vi "4R serial robot 3D simulation.vi"() -> ()   [LabVIEW 2014]
doc: "This example shows a robotic arm with four revolute joints (a 4R serial robot), and demonstrates how to use custom equations to deterministically compute inverse kinematics for the arm."
uses:
  <vilib>/Platform/TimedLoop/XDataNode/timing_clust.ctl
  <vilib>/Platform/TimedLoop/XDataNode/nitl_modes.ctl
  <vilib>/Platform/TimedLoop/XDataNode/wakeup.ctl
  <vilib>/robotics/Kinematics/Plotting/Tree Element.ctl
  <vilib>/robotics/Kinematics/Plotting/Element Type.ctl
  <vilib>/robotics/Kinematics/Plotting/Joint Type.ctl
  <vilib>/Utility/AngleManip/Degrees to Radians (Scalar DBL).vi
  <vilib>/Platform/TimedLoop/XDataNode/XDataNode.xnode
  <vilib>/robotics/Kinematics/Plotting/NI_Robotics_3DKinematics.lvlib
  <vilib>/Platform/TimedLoop/XDataNode/XDNodeRunTimeDep.lvlib
  <vilib>/Utility/AngleManip/NI_AngleManipulation.lvlib
panel:
  out "Invalid Position":bool
  in  "Joint angles":dbl[](array[numeric])
  in  "Y":dbl(slide)=4.790575916230366 scale=-5.0..12.0
  in  "X":dbl(slide)=4.08910891089109 scale=-5.0..12.0
  in  "theta":dbl(knob) scale=-180.0..180.0
  in  "stop":bool
  out "3D Picture Control":refnum<vi>(3d-picture)
  # "This example shows a robotic arm with four revolute joints (a 4R serial robot), and demonstrates how to use custom equations to deterministically compute inverse kinematics for the arm.\n\nUse the X and Y sliders to move the end effector, and the dial to set the rotation of the base. This VI uses inverse kinematics to compute the positions and angles of the joints."
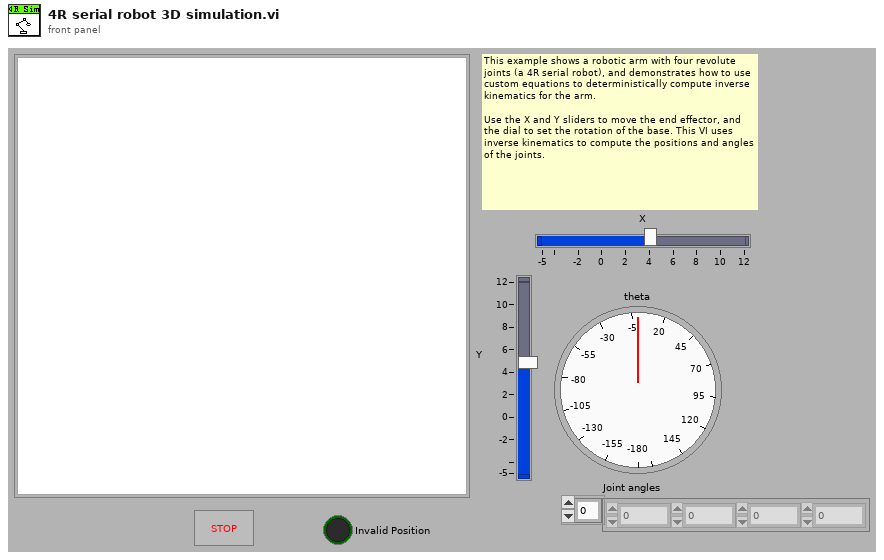
[diagram p1: front panel]
types:
  T1 = typedef "NI_Robotics_3DKinematics.lvlib/Tree Element.ctl" = cluster{"Name":string, "Parent":string, "Type":T2, "Visible?":bool, "Geometry Definition":dbl[], "Position WRT Parent (X,Y,Z)":dbl[], "Rotation WRT Parent (degrees)":dbl[], "Joint Type":T3, "Geometry File Path":path, "Indent Level":i32, "Color":u32}
  T2 = typedef "NI_Robotics_3DKinematics.lvlib/Element Type.ctl" = enum16{"Joint", "Box", "Cylinder", "Cone", "Sphere", "ASE File", "VRML File", "STL File", "Space"}
  T3 = typedef "NI_Robotics_3DKinematics.lvlib/Joint Type.ctl" = enum16{"Trans_X", "Trans_Y", "Trans_Z", "Rot_X", "Rot_Y", "Rot_Z", "None"}
  T4 = typedef "XDNodeRunTimeDep.lvlib/timing_clust.ctl" = cluster{"Expected End [f-1]":u64, "Actual End [f-1]":u64, "Finished Late? [f-1]":bool, "Expected End [i-1]":u64, "Actual End [i-1]":u64, "Finished Late? [i-1]":bool, "Expected Start [i]":u64, "Actual Start [i]":u64, "Expected Start [f]":u64, "Actual Start [f]":u64, "Source Name":string, "Structure Name":string, "Period":i64, "Deadline":i64, "Offset":i64, "Start":i64, "Priority":i32, "Timeout":i32, "Mode":T5, "Wakeup Reason":T6, "Error":errorcluster, "Source Type":string, "Secondary Source Type":string, "Global End Time":u64, "Global Start Time":u64, "Frame Duration":u64, "Iteration Duration":u64, "Assigned CPU":i32, "I/O Scan Engine Mode":u32}
  T5 = typedef "XDNodeRunTimeDep.lvlib/nitl_modes.ctl" = enum32{"No Change", "Process missed periods, maintain original phase", "Discard missed periods, maintain original phase", "Process missed periods, ignore original phase", "Discard missed periods, ignore original phase"}
  T6 = typedef "XDNodeRunTimeDep.lvlib/wakeup.ctl" = enum32{"Normal", "Aborted", "Asynchronous wakeup", "Timing source error", "Timed loop error", "Timeout"}
  T7 = typedef "NI_Robotics_3DKinematics.lvlib/Joint Control.ctl" = cluster{"Joint Refnum":refnum<vi>, "Joint Type":T3, "Position WRT Parent":dbl[], "Rotation WRT Parent":dbl[], "Bar Refnum":refnum<vi>}
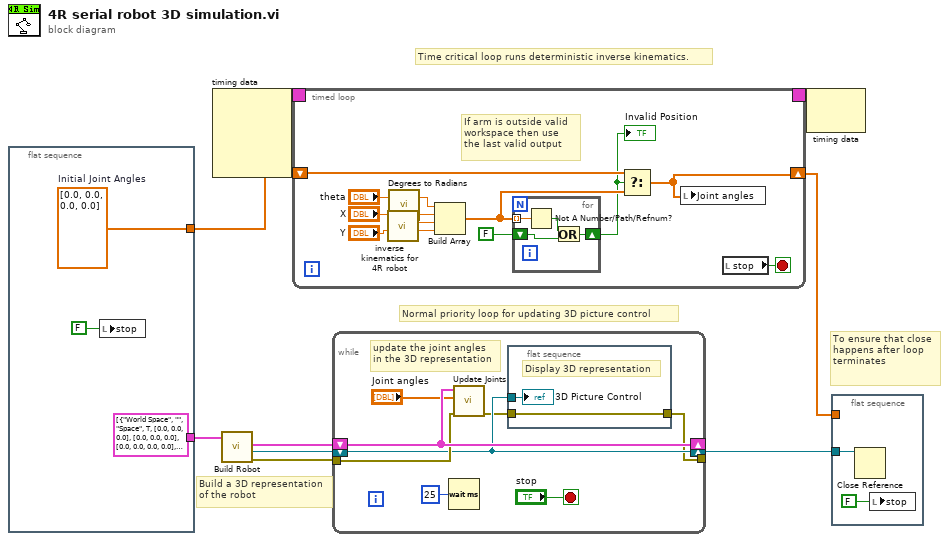
[diagram p0: block diagram]
diagram:
  # "To ensure that close happens after loop terminates"
  # "Build a 3D representation\nof the robot"
  # "Normal priority loop for updating 3D picture control"
  # "Time critical loop runs deterministic inverse kinematics."
  n1 = flat-sequence {
    tunnel: [w12] -> w3
    tunnel: [T1[] [{"Name"="World Space", "Parent"="", "Type"=enum."Space", "Visible?"=TRUE, "Geometry Definition"=[0.0, 0.0, 0.0], "Position WRT Parent (X,Y,Z)"=[0.0, 0.0, 0.0], "Rotation WRT Parent (degrees)"=[0.0, 0.0, 0.0, 0.0], "Joint Type"=enum."None", "Geometry File Path"=path "", "Indent Level"=0, "Color"=16711680}, {"Name"="Base", "Parent"="World Space", "Type"=enum."Cylinder", "Visible?"=TRUE, "Geometry Definition"=[1.0, 1.0, 1.0], "Position WRT Parent (X,Y,Z)"=[0.0, 0.5, 0.0], "Rotation WRT Parent (degrees)"=[1.0, 0.0, 0.0, 90.0], "Joint Type"=enum."None", "Geometry File Path"=path "", "Indent Level"=1, "Color"=16777224}, {"Name"="Joint 1", "Parent"="World Space", "Type"=enum."Joint", "Visible?"=TRUE, "Geometry Definition"=[0.0, 0.0, 0.0], "Position WRT Parent (X,Y,Z)"=[0.0, 1.0, 0.0], "Rotation WRT Parent (degrees)"=[0.0, 0.0, 0.0, 90.0], "Joint Type"=enum."Rot_Y", "Geometry File Path"=path "", "Indent Level"=1, "Color"=16711680}, {"Name"="Joint 3", "Parent"="Joint 1", "Type"=enum."Joint", "Visible?"=TRUE, "Geometry Definition"=[0.0, 0.0, 0.0], "Position WRT Parent (X,Y,Z)"=[0.0, 0.0, 0.0], "Rotation WRT Parent (degrees)"=[0.0, 0.0, 1.0, -90.0], "Joint Type"=enum."Rot_Z", "Geometry File Path"=path "", "Indent Level"=2, "Color"=16711680}, {"Name"="Link 1 A", "Parent"="Joint 3", "Type"=enum."Box", "Visible?"=TRUE, "Geometry Definition"=[0.9, 5.0, 0.5], "Position WRT Parent (X,Y,Z)"=[0.0, 2.0, 0.5], "Rotation WRT Parent (degrees)"=[0.0, 0.0, 0.0, 0.0], "Joint Type"=enum."None", "Geometry File Path"=path "", "Indent Level"=3, "Color"=16711680}, {"Name"="Link 1 B", "Parent"="Joint 3", "Type"=enum."Box", "Visible?"=TRUE, "Geometry Definition"=[0.9, 5.0, 0.5], "Position WRT Parent (X,Y,Z)"=[0.0, 2.0, -0.5], "Rotation WRT Parent (degrees)"=[0.0, 0.0, 0.0, 0.0], "Joint Type"=enum."None", "Geometry File Path"=path "", "Indent Level"=3, "Color"=16711680}, {"Name"="Joint 4", "Parent"="Joint 3", "Type"=enum."Joint", "Visible?"=TRUE, "Geometry Definition"=[0.0, 0.0, 0.0], "Position WRT Parent (X,Y,Z)"=[0.0, 4.0, 0.0], "Rotation WRT Parent (degrees)"=[1.0, 0.0, 0.0, 0.0], "Joint Type"=enum."Rot_Z", "Geometry File Path"=path "", "Indent Level"=3, "Color"=16711680}, {"Name"="Link 2", "Parent"="Joint 4", "Type"=enum."Box", "Visible?"=TRUE, "Geometry Definition"=[0.9, 5.0, 0.5], "Position WRT Parent (X,Y,Z)"=[0.0, 2.0, 0.0], "Rotation WRT Parent (degrees)"=[0.0, 0.0, 0.0, 0.0], "Joint Type"=enum."None", "Geometry File Path"=path "", "Indent Level"=4, "Color"=16711680}, {"Name"="Joint 5", "Parent"="Joint 4", "Type"=enum."Joint", "Visible?"=TRUE, "Geometry Definition"=[0.0, 0.0, 0.0], "Position WRT Parent (X,Y,Z)"=[0.0, 4.0, 0.0], "Rotation WRT Parent (degrees)"=[1.0, 0.0, 0.0, 0.0], "Joint Type"=enum."Rot_Z", "Geometry File Path"=path "", "Indent Level"=4, "Color"=16711680}, {"Name"="Lower Arm 1", "Parent"="Joint 5", "Type"=enum."Box", "Visible?"=TRUE, "Geometry Definition"=[0.9, 4.5, 0.5], "Position WRT Parent (X,Y,Z)"=[0.0, 1.75, 0.5], "Rotation WRT Parent (degrees)"=[0.0, 0.0, 0.0, 0.0], "Joint Type"=enum."None", "Geometry File Path"=path "", "Indent Level"=5, "Color"=16711680}, {"Name"="Lower Arm 2", "Parent"="Joint 5", "Type"=enum."Box", "Visible?"=TRUE, "Geometry Definition"=[0.9, 4.5, 0.5], "Position WRT Parent (X,Y,Z)"=[0.0, 1.75, -0.5], "Rotation WRT Parent (degrees)"=[0.0, 0.0, 0.0, 0.0], "Joint Type"=enum."None", "Geometry File Path"=path "", "Indent Level"=5, "Color"=16711680}, {"Name"="Hand", "Parent"="Joint 5", "Type"=enum."Cylinder", "Visible?"=TRUE, "Geometry Definition"=[1.0, 0.375, 1.0], "Position WRT Parent (X,Y,Z)"=[0.0, 4.0, 0.0], "Rotation WRT Parent (degrees)"=[0.0, 1.0, 0.0, 0.0], "Joint Type"=enum."None", "Geometry File Path"=path "", "Indent Level"=5, "Color"=16711680}, {"Name"="TCF", "Parent"="Joint 5", "Type"=enum."Cylinder", "Visible?"=TRUE, "Geometry Definition"=[0.4, 0.2, 0.1], "Position WRT Parent (X,Y,Z)"=[0.0, 4.5, 0.0], "Rotation WRT Parent (degrees)"=[1.0, 0.0, 0.0, 90.0], "Joint Type"=enum."None", "Geometry File Path"=path "", "Indent Level"=5, "Color"=16776960}]] -> w2
    frame #0 {
      w12 = dbl[] [0.0, 0.0, 0.0, 0.0]  # Initial Joint Angles
      n2 = local write "stop"(FALSE ("stop")) -> ()
    }
  }
  n3 = node-c288() -> (w5:T4)  [unwired: 4 in]
  n4 = call <vilib>:"Build Robot.vi"("Robot Elements"=w2) -> ("error out"=w6:errorcluster, "Scene Out"=w8:refnum<vi>, "Joint Array"=w7:T7[])  [unwired: 8 in]
  n5 = timed-loop {
    timing: w5 -> [_]
    timing-out: [_] -> w4
    shift-right: [w17] -> w1
    shift-left: w3 -> [w18]
    stop <- w16 stop-if-true
    # "If arm is outside valid \nworkspace then use \nthe last valid output"
    n6 = call "inverse kinematics for 4R robot.vi"("y"="Y", "x"="X") -> ("theta3"=w13:dbl, "theta2"=w21:dbl, "theta1"=w22:dbl)  [unwired: 3 in]
    n7 = call-poly <vilib>:"Degrees to Radians.vi"("angle (deg)"="theta") -> ("angle (rad)"=w23:dbl)  [unwired: 2 in]
    n8 = Build Array(w23, w22, w21, w13) -> (w19:dbl[])
    n9 = for {
      tunnel: w19 -> [w29] mode=indexing
      shift-right: [w27] -> w15
      shift-left: FALSE -> [w26]
      n10 = Not A Number/Path/Refnum?(number/path/refnum=w29) -> (NaN/Path/Refnum?=w28:bool)
      n11 = Or(x=w28, y=w26) -> (x .or. y?=w27:bool)
    }
    "Invalid Position" <- w15
    n12 = Select(t=w18, s=w15, f=w19) -> (s? t:f=w17:dbl[])
    n13 = local write "Joint angles"(w17) -> ()
    n14 = local read "stop"() -> (w16:bool)
  }
  n15 = while {
    tunnel: w6 -> [w37]
    shift-right: [w36] -> w9
    shift-left: w8 -> [w36]
    shift-right: [w38] -> _
    shift-left: w7 -> [w38]
    tunnel: [w34] -> _
    stop <- "stop" stop-if-true
    # "update the joint angles\nin the 3D representation"
    n16 = Wait (ms)(milliseconds to wait=u32 25) -> ()  [unwired: 1 out]
    n17 = call <vilib>:"Update Joints.vi"("error in (no error)"=w37, "Joints"="Joint angles", "Joint Array"=w38) -> ("error out"=w35:errorcluster)  [unwired: 8 in]
    n18 = flat-sequence {
      tunnel: w36 -> [w41]
      tunnel: w35 -> [w40]
      tunnel: [w40] -> w34
      frame #0 {
        # "Display 3D representation"
        "3D Picture Control" <- w41
      }
    }
  }
  n19 = node-c288(w4) -> ()  [unwired: 1 out]
  n20 = flat-sequence {
    tunnel: w9 -> [w43]
    tunnel: w1 -> [_]
    frame #0 {
      n21 = Close Reference(reference=w43) -> ()  [unwired: 1 in, 1 out]
      n22 = local write "stop"(FALSE ("stop")) -> ()
    }
  }
